vi "BluetoothReadStringHOST.vi"(9 "Mailbox":T2 items=["Mailbox 1", "Mailbox 2", "Mailbox 3", "Mailbox 4", "Mailbox 5", "Mailbox 6", "Mailbox 7", "Mailbox 8", "Mailbox 9", "Mailbox 10"]) -> (3 "Message":string, 11 "NXT":T1={"Hardware"="NXT", "Flattened String"=""})   [LabVIEW 2010]
uses:
  <vilib>/NXT/Block Support/NXT_MessageMailbox.ctl
  <vilib>/NXT/Subs/LVHSConnector.ctl
panel:
  in  "NXT 2":T1={"Hardware"="NXT", "Flattened String"=""} caption="NXT"
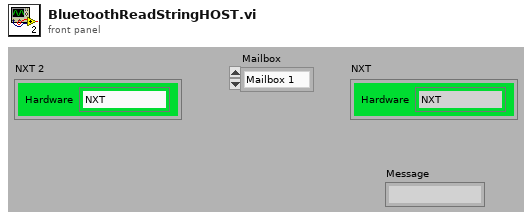
[diagram p1: front panel]
types:
  T1 = typedef "LVHSConnector.ctl" = cluster{"Hardware":string, "Flattened String":string}
  T2 = typedef "NXT_MessageMailbox.ctl" = u8
  T3 = typedef "nxt.ctl" = cluster{"nxtHandle":u32, "fileHandle":u32, "fileIterHandle":u32, "moduleHandle":u32, "modIterHandle":u32, "nxtIterHandle":u32}
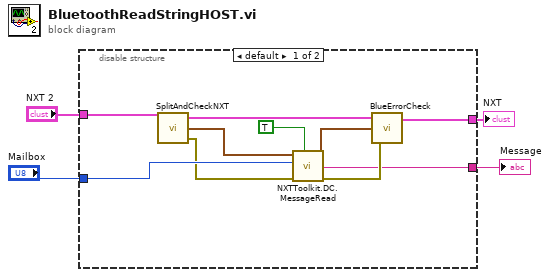
[diagram p0: block diagram]
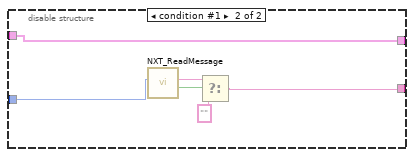
[diagram p2: hidden frame]
diagram:
  n1 = disable-structure shown="default" {
    disable-tunnel: [w11 w16] -> w4
    disable-tunnel: "Mailbox" -> [w8 w17]
    disable-tunnel: [w6 w15] -> w2
    disable-tunnel: "NXT 2" -> [w5 w15]
    frame condition #0 (active) {
      n2 = call <vilib>:"SplitAndCheckNXT.vi"("NXT"=w5) -> ("NXT"=w14:T1, "NXTObject out"=w9:T3, "error out"=w7:errorcluster)  [unwired: 1 in]
      n3 = call <vilib>:"NXTToolkit.DC.MessageRead.vi"("Read Master's inbox (T)"=TRUE, "error in (no error)"=w7, "Mailbox (Mailbox 1)"=w8, "NXTObject"=w9) -> ("error out"=w12:errorcluster, "Message"=w11:string, "NXTObject dup"=w13:T3)  [unwired: 1 in, 4 out]
      n4 = call <vilib>:"BlueErrorCheck.vi"("error in"=w12, "NXTObject"=w13, "NXT"=w14) -> ("NXT"=w6:T1)  [unwired: 1 out]
    }
    frame condition #1 {
      n5 = call <vilib>:"NXT_ReadMessage.vi"("Mailbox"=w17) -> ("Message Received"=w20:bool, "Text out"=w19:string)  [unwired: 1 in, 8 out]
      n6 = Select(t=w19, s=w20, f="") -> (s? t:f=w16:string)
    }
  }
  "Message" <- w4
  "NXT" <- w2
